vi "SOLICITAR BASE DE DATOS.vi"(8 "error in (no error)":errorcluster, 10 "BASE DE DATOS":string, 11 "DATABASE_MANEJO in":refnum<class "DATABASE_MANEJO.lvclass">) -> (0 "error out":errorcluster, 3 "DATABASE_MANEJO out":refnum<class "DATABASE_MANEJO.lvclass">)   [LabVIEW 2019, in "DATABASE_MANEJO.lvlib" / "DATABASE_MANEJO.lvclass"]
uses:
  DATABASE_MANEJO.lvclass
  DATABASE_MANEJO.lvclass/DATABASE_MANEJO.ctl
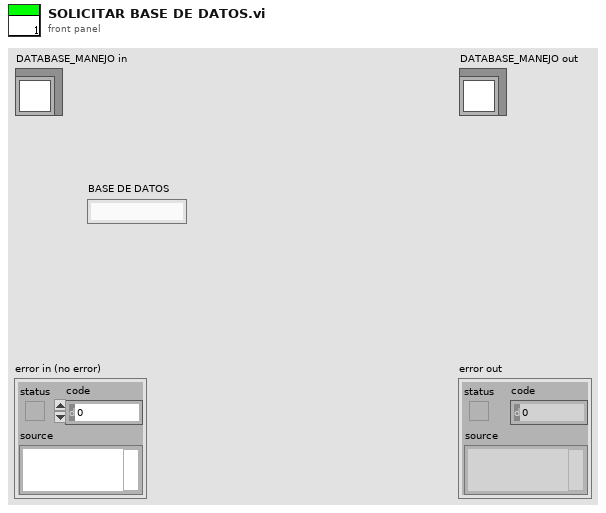
[diagram p1: front panel]
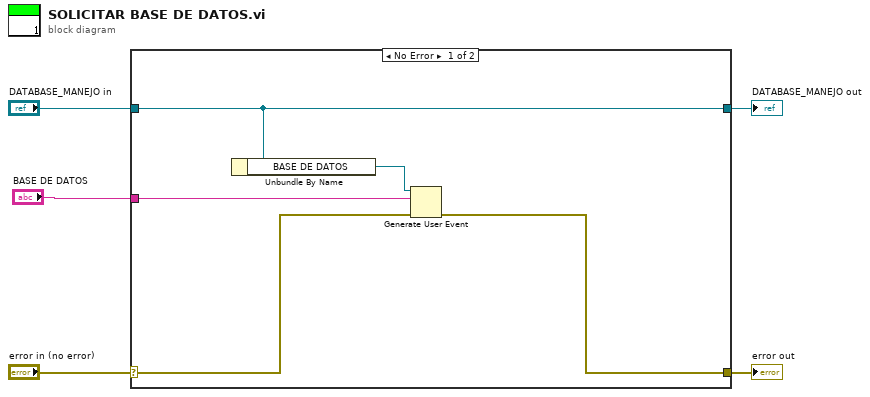
[diagram p0: block diagram]
diagram:
  n1 = case shown="No Error" "error in (no error)" {
    selector: "error in (no error)" -> [w7 w12]
    tunnel: [w6 w12] -> w4
    tunnel: [w10 w11] -> w2
    tunnel: "DATABASE_MANEJO in" -> [w10 w11]
    tunnel: "BASE DE DATOS" -> [w8 _]
    frame No Error {
      n2 = Unbundle By Name(w10) -> ("BASE DE DATOS"=w9:refnum<user-event>)
      n3 = Generate User Event(user event=w9, event data cluster=w8, error in=w7) -> (error out=w6:errorcluster)  [unwired: 1 in, 1 out]
    }
    frame Error {
    }
  }
  "error out" <- w4
  "DATABASE_MANEJO out" <- w2
